vi "testIncrement.vi"() -> ()   [LabVIEW 2012]
panel:
  in  "Cluster 2":T1
  in  "Cluster":T2
  in  "stop":bool
  in  "Timing Sequence":T3(array[cluster])=[{"Active"=TRUE, "counter"="PXI1Slot9/ctr7", "Units Dt"="ns", "Units Time"="ns", "Channel Name"="", "Time"=0.0, "Pulse Width"=0.0, "Units Width"="ns", "Increment"="Off", "Dt"=0.0, "-"=FALSE}] {"Dt" format="%_3g"; "Pulse Width" format="%_3g"; "Time" format="%_3g"}
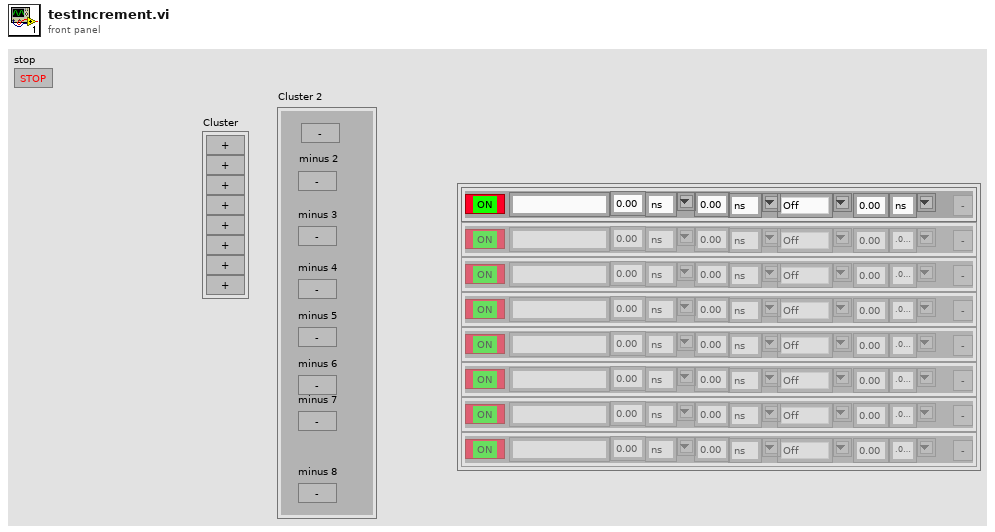
[diagram p1: front panel]
types:
  T1 = cluster{"minus 1":bool, "minus 2":bool, "minus 3":bool, "minus 4":bool, "minus 5":bool, "minus 6":bool, "minus 7":bool, "minus 8":bool}
  T2 = cluster{"plus 1":bool, "plus 2":bool, "plus 3":bool, "plus 4":bool, "plus 5":bool, "plus 6":bool, "plus 7":bool, "plus 8":bool}
  T3 = cluster{"Active":bool, "counter":tag, "Units Dt":string, "Units Time":string, "Channel Name":string, "Time":dbl, "Pulse Width":dbl, "Units Width":string, "Increment":string, "Dt":dbl, "-":bool}[]
  T4 = cluster{"Active":bool, "counter":tag, "Units Dt":string, "Units Time":string, "Channel Name":string, "Time":dbl, "Pulse Width":dbl, "Units Width":string, "Increment":string, "Dt":dbl, "-":bool}
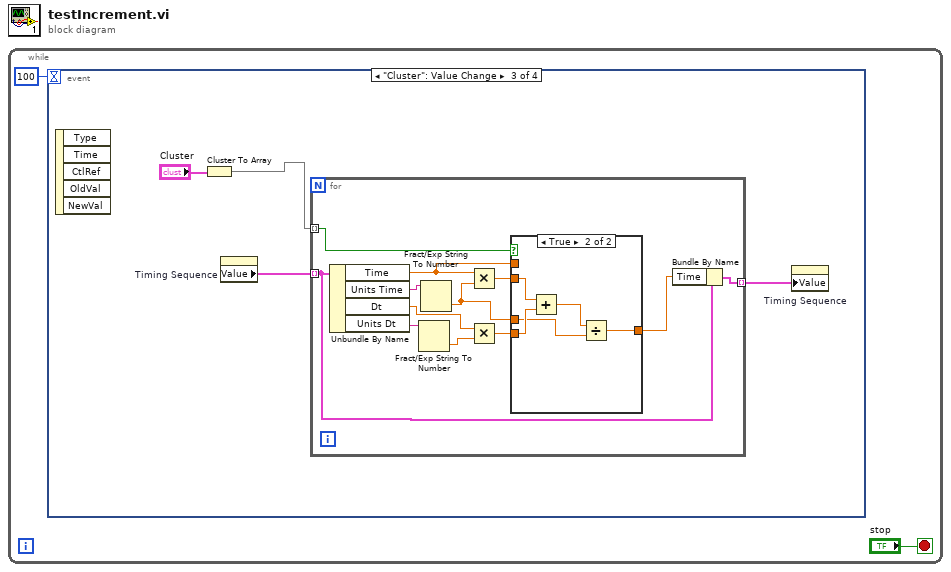
[diagram p0: block diagram]
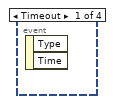
[diagram p2: hidden frame]
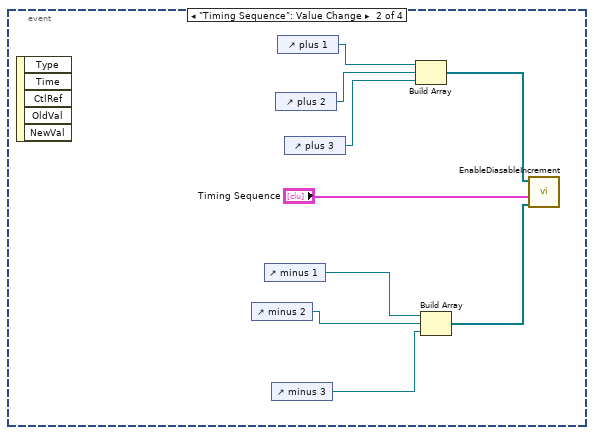
[diagram p3: hidden frame]
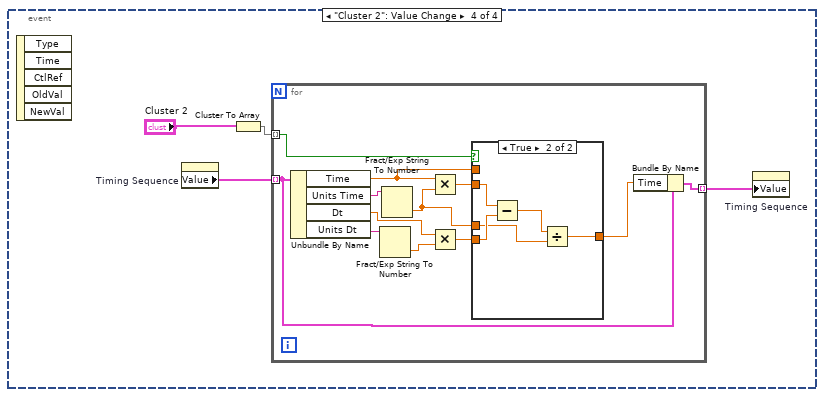
[diagram p5: hidden frame]
diagram:
  n1 = while {
    stop <- "stop" stop-if-true
    n2 = event shown="[2] \"Cluster\": Value Change" {
      selector: _ -> [_ _ _ _]
      dyn-events: _ -> [_ _ _ _]
      timeout: 100 -> [_ _ _ _]
      event Timeout {
        n3 = event-data() -> ()  [unwired: 1 in, 2 out]
      }
      event "Timing Sequence": Value Change {
        n4 = event-data() -> ()  [unwired: 1 in, 5 out]
        n5 = control-ref of="minus 2"() -> (w5:refnum<vi>)
        n6 = control-ref of="minus 1"() -> (w4:refnum<vi>)
        n7 = control-ref of="minus 3"() -> (w3:refnum<vi>)
        n8 = control-ref of="plus 2"() -> (w9:refnum<vi>)
        n9 = control-ref of="plus 1"() -> (w10:refnum<vi>)
        n10 = control-ref of="plus 3"() -> (w8:refnum<vi>)
        n11 = Build Array(w10, w9, w8) -> (w7:refnum<vi>[])
        n12 = Build Array(w4, w5, w3) -> (w6:refnum<vi>[])
        n13 = call "EnableDiasableIncrement.vi"("appended array 2"=w6, "NewVal"="Timing Sequence", "appended array"=w7) -> ()  [unwired: 9 in]
      }
      event "Cluster": Value Change {
        n14 = event-data() -> ()  [unwired: 1 in, 5 out]
        n15 = Cluster To Array(cluster="Cluster") -> (array=w12:bool[])
        n16 = property on="Timing Sequence" class="Arr (strict)"() -> ("Value"=w15:T3)  [unwired: 2 in, 2 out]
        n17 = for {
          tunnel: w15 -> [w23] mode=indexing
          tunnel: w12 -> [w27] mode=indexing
          tunnel: [w22] -> w14 mode=indexing
          n18 = Unbundle By Name(w23) -> ("Time"=w20:dbl, "Units Time"=w17:string, "Dt"=w26:dbl, "Units Dt"=w19:string)
          n19 = Fract/Exp String To Number(string=w19) -> (number=w18:dbl)  [unwired: 3 in, 1 out]
          n20 = Fract/Exp String To Number(string=w17) -> (number=w16:dbl)  [unwired: 3 in, 1 out]
          n21 = Multiply(x=w20, y=w16) -> (x*y=w25:dbl)
          n22 = Multiply(x=w26, y=w18) -> (x*y=w24:dbl)
          n23 = case shown="True" w27 {
            tunnel: w25 -> [_ w33]
            tunnel: w24 -> [_ w32]
            tunnel: w16 -> [_ w30]
            tunnel: [w28 w29] -> w21
            tunnel: w20 -> [w28 _]
            frame False {
            }
            frame True {
              n24 = Add(x=w33, y=w32) -> (x+y=w31:dbl)
              n25 = Divide(x=w31, y=w30) -> (x/y=w29:dbl)
            }
          }
          n26 = Bundle By Name(cluster=w23, "Time"=w21) -> (w22:T4)
        }
        n27 = property on="Timing Sequence" class="Arr (strict)"("Value"=w14) -> ()  [unwired: 2 in, 2 out]
      }
      event "Cluster 2": Value Change {
        n28 = event-data() -> ()  [unwired: 1 in, 5 out]
        n29 = property on="Timing Sequence" class="Arr (strict)"() -> ("Value"=w37:T3)  [unwired: 2 in, 2 out]
        n30 = Cluster To Array(cluster="Cluster 2") -> (array=w36:bool[])
        n31 = for {
          tunnel: w37 -> [w45] mode=indexing
          tunnel: w36 -> [w49] mode=indexing
          tunnel: [w44] -> w35 mode=indexing
          n32 = Unbundle By Name(w45) -> ("Time"=w42:dbl, "Units Time"=w39:string, "Dt"=w48:dbl, "Units Dt"=w41:string)
          n33 = Fract/Exp String To Number(string=w41) -> (number=w40:dbl)  [unwired: 3 in, 1 out]
          n34 = Fract/Exp String To Number(string=w39) -> (number=w38:dbl)  [unwired: 3 in, 1 out]
          n35 = Multiply(x=w42, y=w38) -> (x*y=w47:dbl)
          n36 = Multiply(x=w48, y=w40) -> (x*y=w46:dbl)
          n37 = case shown="True" w49 {
            tunnel: w47 -> [_ w55]
            tunnel: w46 -> [_ w54]
            tunnel: w38 -> [_ w52]
            tunnel: [w50 w51] -> w43
            tunnel: w42 -> [w50 _]
            frame False {
            }
            frame True {
              n38 = Subtract(x=w55, y=w54) -> (x-y=w53:dbl)
              n39 = Divide(x=w53, y=w52) -> (x/y=w51:dbl)
            }
          }
          n40 = Bundle By Name(cluster=w45, "Time"=w43) -> (w44:T4)
        }
        n41 = property on="Timing Sequence" class="Arr (strict)"("Value"=w35) -> ()  [unwired: 2 in, 2 out]
      }
    }
  }
